vi "Get Decimation.vi"(11 "Timing in":refnum<class "Timing.lvclass">) -> (2 "Decimation":u64=1, 3 "Timing out":refnum<class "Timing.lvclass">)   [LabVIEW 2019, in "DSF Core.lvlib" / "Timing.lvclass"]
uses:
  Timing.lvclass
  Timing.lvclass/Timing.ctl
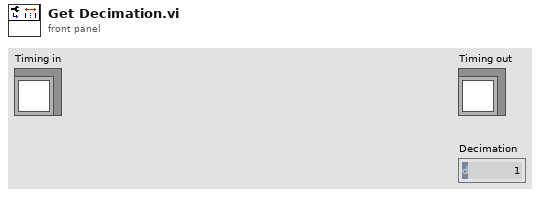
[diagram p1: front panel]
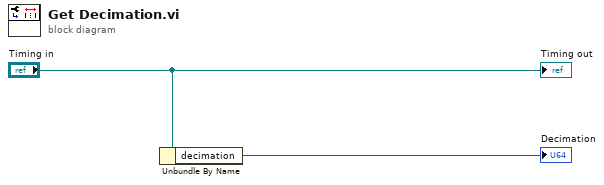
[diagram p0: block diagram]
diagram:
  n1 = Unbundle By Name("Timing in") -> ("decimation"=→"Decimation":u64)
  "Timing out" <- "Timing in"
